vi "Configure.vi"(8 "error in (no error)":errorcluster, 11 "Tomo in":refnum<class "Tomo.lvclass">) -> (0 "error out":errorcluster, 2 "cancelled?":bool, 3 "Tomo out":refnum<class "Tomo.lvclass">)   [LabVIEW 2012, in "Tomo.lvclass"]
doc: "The configure method configures the details for the RabbitMQ connection. \n\nIn the derived class, make a call to the parent for setting these parameters."
uses:
  Tomo.lvclass
  <vilib>/Utility/miscctls.llb/LVPointTypeDef.ctl
  Tomo.lvclass/Tomo.ctl
  <vilib>/Distrio/Murmex/Murmex/Murmex.lvclass
panel:
  in  "Tab Control":enum32{"Slave components", "Other", "Pre-tomo"}(tab)
  in  "Waveform component":string
  in  "Pretomo camera component":string
  in  "Orca - Slave component":string
  in  "Stack component":string
  in  "Orca - Master component":string
  in  "Stages component":string
  in  "Autofocus component":string
  in  "AOTF component":string
  in  "resolution":dbl
  in  "lateral magnification":dbl
  in  "Orca pixel size":dbl[unit]
  in  "mapping file folder":path
  in  "default stages speed":dbl[unit]
  in  "stack overhead time":dbl[unit]
  in  "camera pixel size":dbl[unit]=0.00039999999999999996
  in  "camera y res":u32
  in  "camera x res":u32
  in  "small images base path":path
  in  "full image base path":path
  in  "offset centres":dbl[unit]
  in  "pixel size (object space)":dbl[unit]
  in  "downsampling factor":u32
  in  "Z step size":dbl[unit]=2e-06
  in  "X step size":dbl[unit]=0.00039999999999999996
  in  "Y step size":dbl[unit]=0.00039999999999999996
  in  "button::cancel":bool
  in  "button::configure_murmex":bool
  in  "button::ok":bool
  # "Orca camera"
  # "Camera used"
  # "empirically determined values"
  # "Stitching"
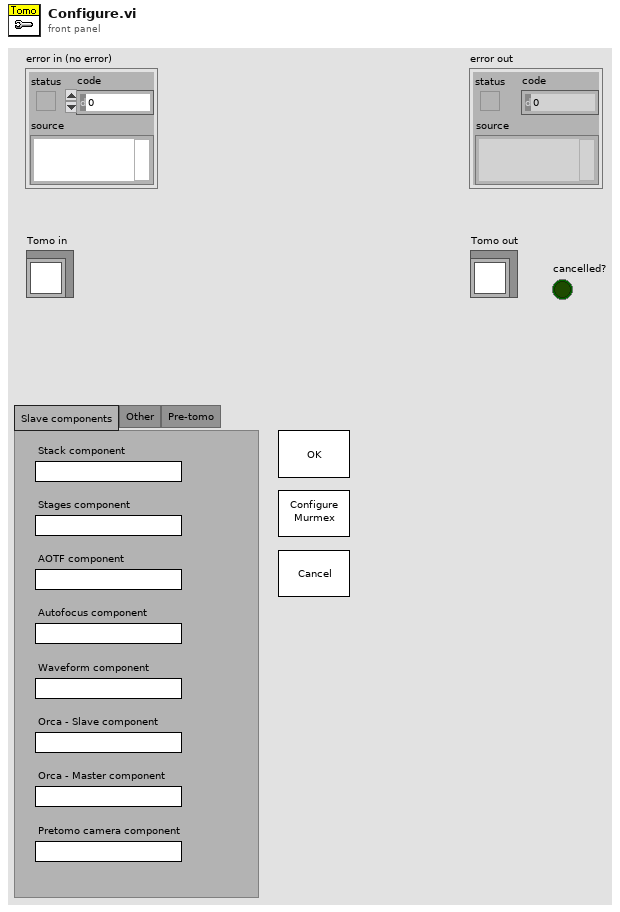
[diagram p1: front panel]
types:
  T1 = typedef "LVPointTypeDef.ctl" = cluster{"Horizontal":i16, "Vertical":i16}
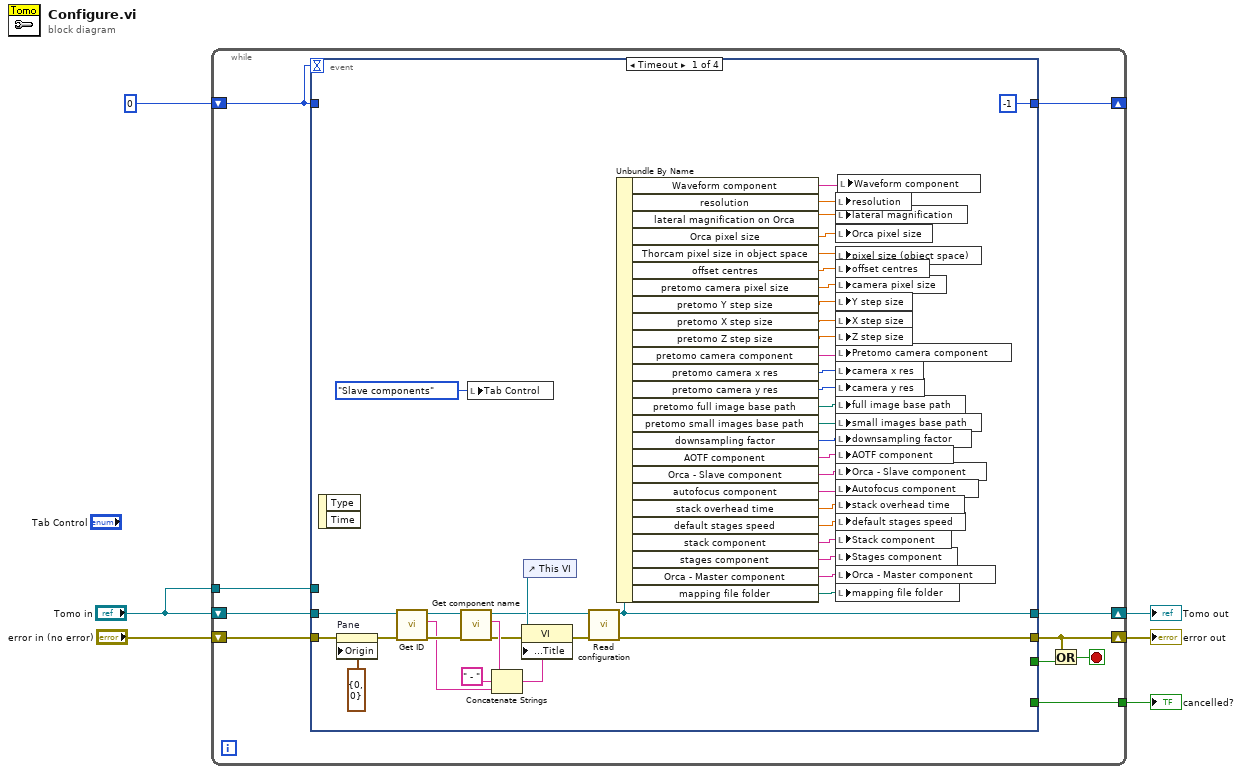
[diagram p0: block diagram]
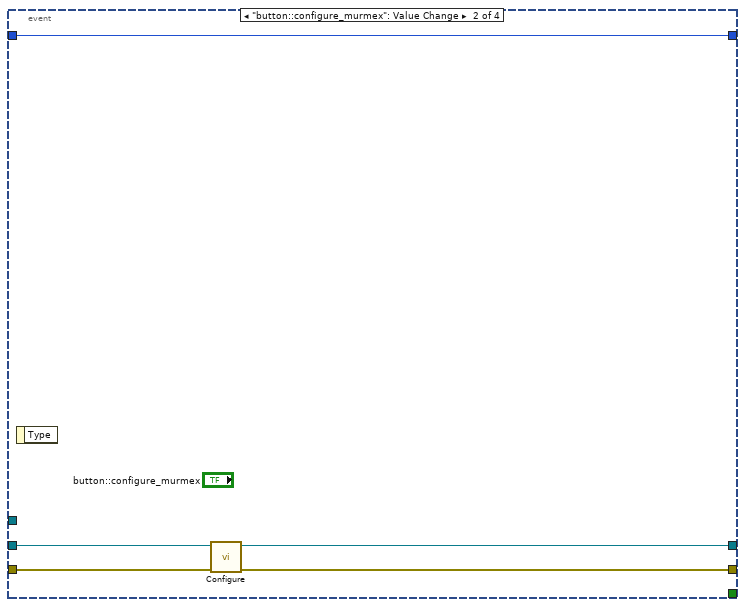
[diagram p2: hidden frame]
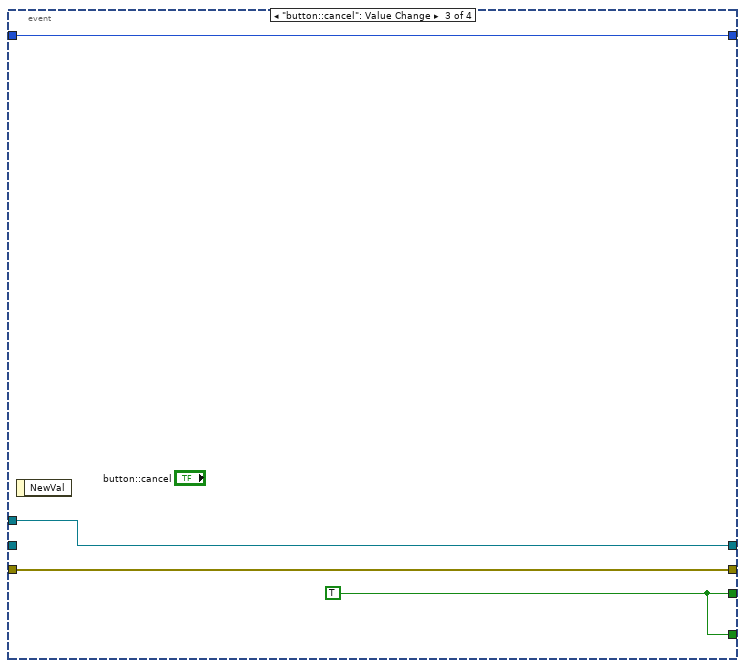
[diagram p3: hidden frame]
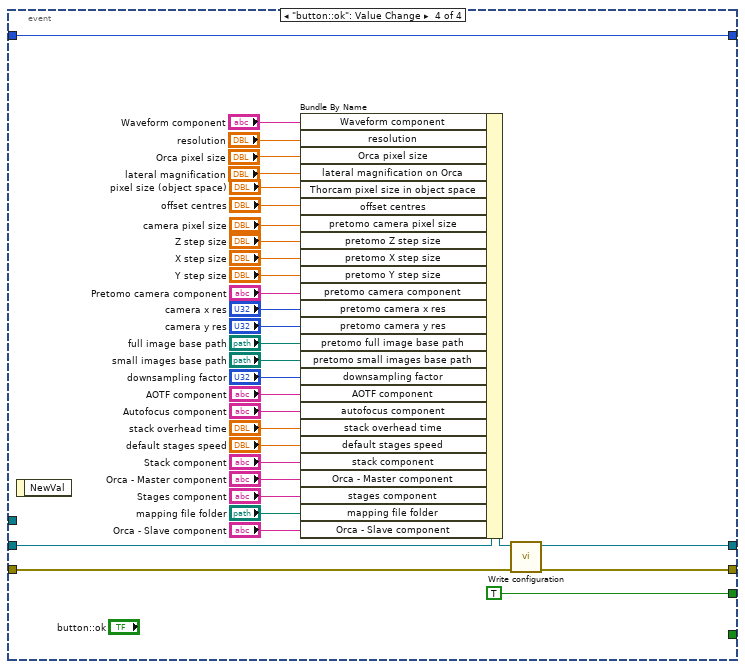
[diagram p4: hidden frame]
diagram:
  n1 = while {
    shift-right: [w9] -> w2
    shift-left: "error in (no error)" -> [w16]
    shift-right: [w12] -> _
    shift-left: 0 -> [w15]
    shift-right: [w11] -> w1
    shift-left: "Tomo in" -> [w14]
    tunnel: "Tomo in" -> [w13]
    tunnel: [w7] -> w3
    stop <- w8 stop-if-true
    n2 = event shown="[0] Timeout" {
      selector: _ -> [_ _ _ _]
      dyn-events: _ -> [_ _ _ _]
      timeout: w15 -> [_ _ _ _]
      tunnel: w16 -> [w59 w64 w67 w96]
      tunnel: w15 -> [_ w60 w65 w100]
      tunnel: w14 -> [w56 w62 _ w95]
      tunnel: w13 -> [_ _ w68 _]
      tunnel: [-1 w60 w65 w100] -> w12
      tunnel: [w43 w61 w68 w97] -> w11
      tunnel: [w44 w63 w67 w99] -> w9
      tunnel: [_ _ w66 TRUE] -> w10
      tunnel: [_ _ w66 _] -> w7
      event Timeout {
        n3 = event-data() -> ()  [unwired: 1 in, 2 out]
        n4 = property on="Pane" class="Pane"(error in=w59, "Origin"=T1 {"Horizontal"=0, "Vertical"=0}) -> (error out=w57:errorcluster)  [unwired: 1 in, 1 out]
        n5 = call <vilib>:"Get ID.vi"("error in (no error)"=w57, "Murmex in"=w56) -> ("error out"=w55:errorcluster, "component id"=w52:string, "Murmex out"=w54:refnum<class "Tomo.lvclass">)  [unwired: 7 in]
        n6 = call <vilib>:"Get component name.vi"("error in (no error)"=w55, "Murmex in"=w54) -> ("error out"=w49:errorcluster, "component name"=w53:string, "Murmex out"=w45:refnum<class "Tomo.lvclass">)  [unwired: 7 in]
        n7 = local write "Tab Control"(enum32{"Slave components", "Other", "Pre-tomo"}."Slave components" ("Tab Control")) -> ()
        n8 = Concatenate Strings(w53, " - " ("string"), w52) -> (w47:string)
        n9 = control-ref of="This VI"() -> (w48:refnum<vi>)
        n10 = property class="VI"(reference=w48, error in=w49, "Front Panel.Title"=w47) -> (error out=w46:errorcluster)  [unwired: 1 out]
        n11 = call <vilib>:"Read configuration.vi"("error in (no error)"=w46, "Murmex in"=w45) -> ("error out"=w44:errorcluster, "Murmex out"=w43:refnum<class "Tomo.lvclass">)  [unwired: 7 in, 1 out]
        n12 = Unbundle By Name(w43) -> ("Waveform component"=w17:string, "resolution"=w18:dbl, "lateral magnification on Orca"=w20:dbl, "Orca pixel size"=w21:dbl[unit], "Thorcam pixel size in object space"=w22:dbl[unit], "offset centres"=w23:dbl[unit], "pretomo camera pixel size"=w26:dbl[unit], "pretomo Y step size"=w27:dbl[unit], "pretomo X step size"=w28:dbl[unit], "pretomo Z step size"=w29:dbl[unit], "pretomo camera component"=w30:string, "pretomo camera x res"=w25:u32, "pretomo camera y res"=w31:u32, "pretomo full image base path"=w33:path, "pretomo small images base path"=w32:path, "downsampling factor"=w24:u32, "AOTF component"=w34:string, "Orca - Slave component"=w35:string, "autofocus component"=w36:string, "stack overhead time"=w38:dbl[unit], "default stages speed"=w37:dbl[unit], "stack component"=w39:string, "stages component"=w40:string, "Orca - Master component"=w41:string, "mapping file folder"=w42:path)
        n13 = local write "resolution"(w18) -> ()
        n14 = local write "lateral magnification"(w20) -> ()
        n15 = local write "Orca pixel size"(w21) -> ()
        n16 = local write "pixel size (object space)"(w22) -> ()
        n17 = local write "offset centres"(w23) -> ()
        n18 = local write "camera pixel size"(w26) -> ()
        n19 = local write "Y step size"(w27) -> ()
        n20 = local write "X step size"(w28) -> ()
        n21 = local write "Z step size"(w29) -> ()
        n22 = local write "Pretomo camera component"(w30) -> ()
        n23 = local write "camera x res"(w25) -> ()
        n24 = local write "camera y res"(w31) -> ()
        n25 = local write "full image base path"(w33) -> ()
        n26 = local write "small images base path"(w32) -> ()
        n27 = local write "downsampling factor"(w24) -> ()
        n28 = local write "AOTF component"(w34) -> ()
        n29 = local write "Orca - Slave component"(w35) -> ()
        n30 = local write "Autofocus component"(w36) -> ()
        n31 = local write "stack overhead time"(w38) -> ()
        n32 = local write "default stages speed"(w37) -> ()
        n33 = local write "Stack component"(w39) -> ()
        n34 = local write "Stages component"(w40) -> ()
        n35 = local write "Orca - Master component"(w41) -> ()
        n36 = local write "mapping file folder"(w42) -> ()
        n37 = local write "Waveform component"(w17) -> ()
      }
      event "button::configure_murmex": Value Change {
        n38 = event-data() -> ()  [unwired: 1 in, 1 out]
        n39 = call-parent "Configure.vi"("error in (no error)"=w64, "Murmex in"=w62) -> ("error out"=w63:errorcluster, "Murmex out"=w61:refnum<class "Tomo.lvclass">)  [unwired: 7 in, 1 out]
      }
      event "button::cancel": Value Change {
        w66 = TRUE
        n40 = event-data() -> ()  [unwired: 1 in, 1 out]
      }
      event "button::ok": Value Change {
        n41 = event-data() -> ()  [unwired: 1 in, 1 out]
        n42 = Bundle By Name(cluster=w95, "Waveform component"="Waveform component", "resolution"="resolution", "Orca pixel size"="Orca pixel size", "lateral magnification on Orca"="lateral magnification", "Thorcam pixel size in object space"="pixel size (object space)", "offset centres"="offset centres", "pretomo camera pixel size"="camera pixel size", "pretomo Z step size"="Z step size", "pretomo X step size"="X step size", "pretomo Y step size"="Y step size", "pretomo camera component"="Pretomo camera component", "pretomo camera x res"="camera x res", "pretomo camera y res"="camera y res", "pretomo full image base path"="full image base path", "pretomo small images base path"="small images base path", "downsampling factor"="downsampling factor", "AOTF component"="AOTF component", "autofocus component"="Autofocus component", "stack overhead time"="stack overhead time", "default stages speed"="default stages speed", "stack component"="Stack component", "Orca - Master component"="Orca - Master component", "stages component"="Stages component", "mapping file folder"="mapping file folder", "Orca - Slave component"="Orca - Slave component") -> (w94:refnum<class "Tomo.lvclass">)
        n43 = call <vilib>:"Write configuration.vi"("error in (no error)"=w96, "Murmex in"=w94) -> ("error out"=w99:errorcluster, "Murmex out"=w97:refnum<class "Tomo.lvclass">)  [unwired: 8 in]
      }
    }
    n44 = Or(x=w9, y=w10) -> (x .or. y?=w8:bool)
  }
  "error out" <- w2
  "Tomo out" <- w1
  "cancelled?" <- w3
